vi "test_ScopeInstrument_CallCreateSessionWithUnregisteredSessionReserved_RemoteSessionCreated.vi"(8 "error in":errorcluster) -> (0 "error out":errorcluster, 2 "result":string, 3 "pass":bool)   [LabVIEW 2020, in "MeasurementServerTests.lvlib"]
uses:
  MeasurementServerTests.lvlib
  Runtime/MeasurementLink niScope/Create Sessions - 1Sess.vi
  Runtime/MeasurementLink niScope/MeasurementLink niScope.lvlib
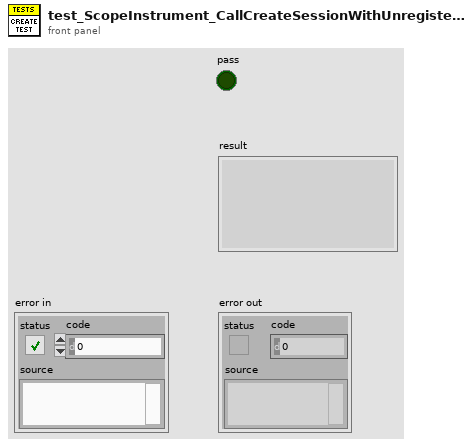
[diagram p1: front panel]
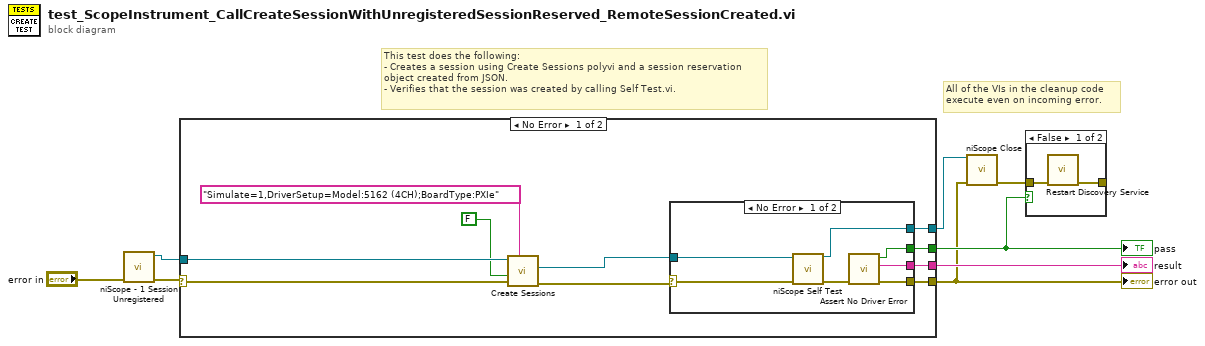
[diagram p0: block diagram]
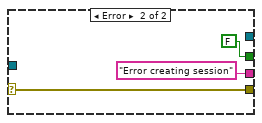
[diagram p2: hidden frame]
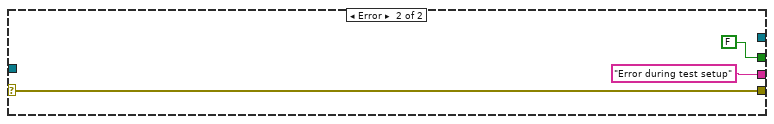
[diagram p3: hidden frame]
diagram:
  # "All of the VIs in the cleanup code\nexecute even on incoming error."
  # "This test does the following:\n- Creates a session using Create Sessions polyvi and a session reservation\nobject created from JSON.\n- Verifies that the session was created by calling Self Test.vi."
  n1 = call "niScope - 1 Session Unregistered.vi"("error in"="error in") -> ("error out"=w2:errorcluster, "Session Reservation out"=w1:refnum<class "Session Reservation.lvclass">)  [unwired: 9 in]
  n2 = case shown="No Error" w2 {
    selector: w2 -> [w12 w29]
    tunnel: [w17 w29] -> w4
    tunnel: [w18 FALSE] -> w5
    tunnel: [w16 "Error during test setup" ("f")] -> w8
    tunnel: [w15 _] -> w7
    tunnel: w1 -> [w11 _]
    frame No Error {
      n3 = call-poly "Create Sessions.vi"("option string"="Simulate=1,DriverSetup=Model:5162 (4CH);BoardType:PXIe", "error in"=w12, "reset"=FALSE, "session reservation in"=w11) -> ("error out"=w10:errorcluster, "session"=w13:refnum<k15>)  [unwired: 4 in, 2 out]
      n4 = case shown="No Error" w10 {
        selector: w10 -> [w19 w27]
        tunnel: [w25 FALSE] -> w18
        tunnel: [w23 w27] -> w17
        tunnel: [w24 "Error creating session"] -> w16
        tunnel: w13 -> [w20 _]
        tunnel: [w22 _] -> w15
        frame No Error {
          n5 = call <instrlib>:"niScope Self Test.vi"("instrument handle"=w20, "error in"=w19) -> ("instrument handle out"=w22:refnum<k15>, "error out"=w21:errorcluster)  [unwired: 10 in, 2 out]
          n6 = call "Assert No Driver Error.vi"("error in"=w21) -> ("error out"=w23:errorcluster, "result"=w24:string, "pass?"=w25:bool)  [unwired: 8 in]
        }
        frame Error {
        }
      }
    }
    frame Error {
    }
  }
  "error out" <- w4
  "pass" <- w5
  "result" <- w8
  n7 = call <instrlib>:"niScope Close.vi"("instrument handle"=w7, "error in"=w4) -> ("error out"=w6:errorcluster)  [unwired: 13 in]
  n8 = case shown="False" w5 {
    tunnel: w6 -> [w33 _]
    tunnel: [w32 _] -> _
    frame False {
      n9 = call "Restart Discovery Service.vi"("error in"=w33) -> ("error out"=w32:errorcluster)  [unwired: 10 in]
    }
    frame True {
    }
  }
